vi "Write lst.vi"(8 "error in (no error)":errorcluster, 10 "ClockTimes.lvclass":refnum<class "ClockTimes.lvclass">, 11 "CurrentTimes in":refnum<class "CurrentTimes.lvclass">) -> (0 "error out":errorcluster, 3 "CurrentTimes out":refnum<class "CurrentTimes.lvclass">)   [LabVIEW 2014, in "TCSDataDefinitions.lvlib" / "TCSPublicStatus.lvlib" / "CurrentTimes.lvlib" / "CurrentTimes.lvclass"]
uses:
  CurrentTimes.lvclass
  ClockTimes/ClockTimes.lvclass
  CurrentTimes.lvclass/CurrentTimes.ctl
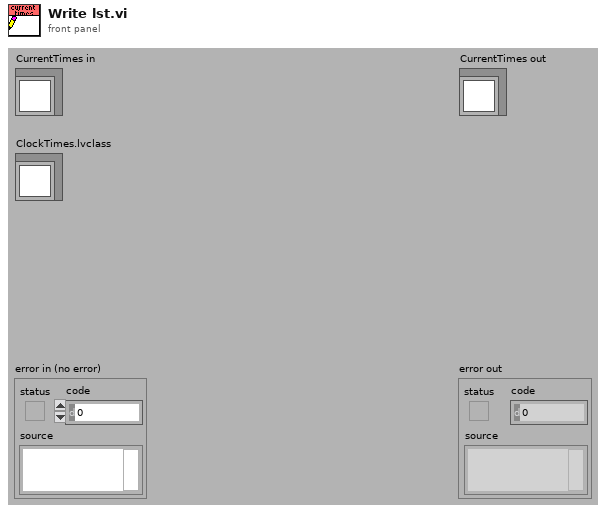
[diagram p1: front panel]
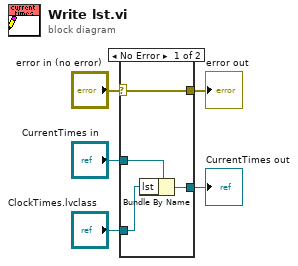
[diagram p0: block diagram]
diagram:
  n1 = case shown="No Error" "error in (no error)" {
    selector: "error in (no error)" -> [w9 w10]
    tunnel: [w9 w10] -> w4
    tunnel: [w7 w11] -> w2
    tunnel: "CurrentTimes in" -> [w8 w11]
    tunnel: "ClockTimes.lvclass" -> [w6 _]
    frame No Error {
      n2 = Bundle By Name(cluster=w8, "lst"=w6) -> (w7:refnum<class "CurrentTimes.lvclass">)
    }
    frame Error {
    }
  }
  "error out" <- w4
  "CurrentTimes out" <- w2
